vi "Enumerate Actions.vi"() -> (2 "Actions":map{string, refnum<class "CLIAction.lvclass">}(c390))   [LabVIEW 2020, in "GPackTools.lvlib"]
uses:
  GPackTools.lvlib
  CLIAction/CLIAction.lvclass
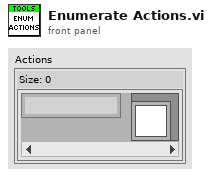
[diagram p1: front panel]
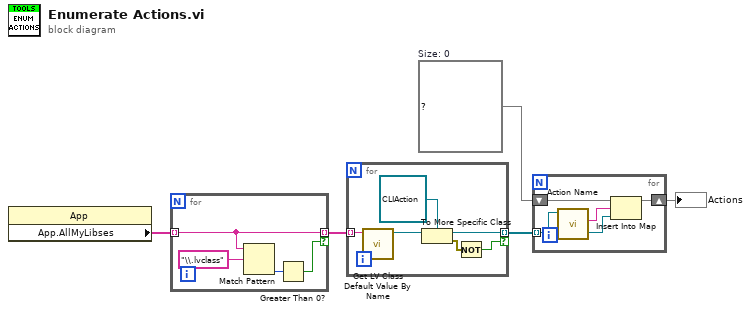
[diagram p0: block diagram]
diagram:
  w2 = map{string, refnum<class "CLIAction.lvclass">} {}  # Size: 0
  n1 = property class="App"() -> ("App.AllMyLibses"=w5:string[])  [unwired: 2 in, 2 out]
  n2 = for {
    tunnel: w5 -> [w8] mode=indexing
    tunnel: [w8] -> w4 mode=indexing if=w6
    n3 = Match Pattern(string=w8, regular expression="\\.lvclass") -> (offset past match=w7:i32)  [unwired: 1 in, 3 out]
    n4 = Greater Than 0?(x=w7) -> (x > 0?=w6:bool)
  }
  n5 = for {
    tunnel: w4 -> [w15] mode=indexing
    tunnel: [w10] -> w3 mode=indexing if=w11
    n6 = call <vilib>:"Get LV Class Default Value By Name.vi"("class name"=w15) -> ("object"=w13:refnum<class>)  [unwired: 9 in, 1 out]
    n7 = To More Specific Class(target class=refnum<class "CLIAction.lvclass"> refnum ("GPackTools.lvlib:CLIAction.lvclass"), reference=w13) -> (specific class reference=w10:refnum<class "CLIAction.lvclass">, error out=w12:errorcluster)  [unwired: 1 in]
    n8 = Not(x=w12) -> (.not. x?=w11:bool)
  }
  n9 = for {
    tunnel: w3 -> [w17] mode=indexing
    shift-right: [w16] -> w1
    shift-left: w2 -> [w19]
    n10 = call-dynamic "Action Name.vi"("CLIAction in"=w17) -> ("Action Name"=w18:string)  [unwired: 10 in]
    n11 = Insert Into Map(map in=w19, key=w18, value=w17) -> (map out=w16:map{string, refnum<class "CLIAction.lvclass">})  [unwired: 2 out]
  }
  "Actions" <- w1
